vi "Post-Build Action.vi"(5 "Files Generated by Build":path[](array[path]), 6 "Top Level/Always Included VIs":path[](array[path]), 7 "Destination Path":path, 8 "error in":errorcluster, 9 "Target Name":string, 10 "Build Specification Name":string, 11 "Project Path":path) -> (0 "error out":errorcluster)   [LabVIEW 2026]
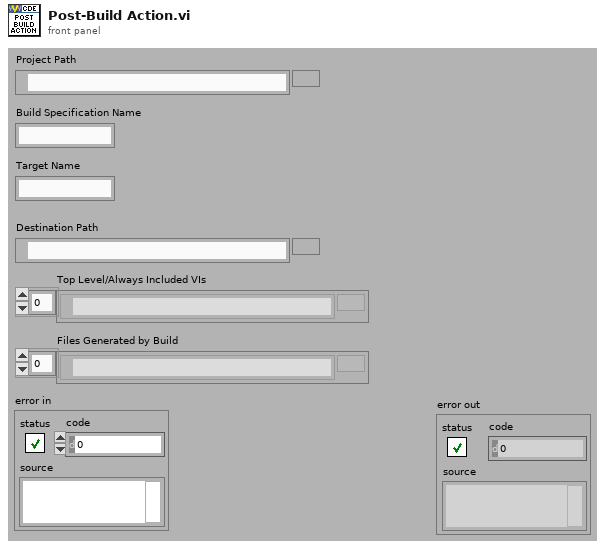
[diagram p1: front panel]
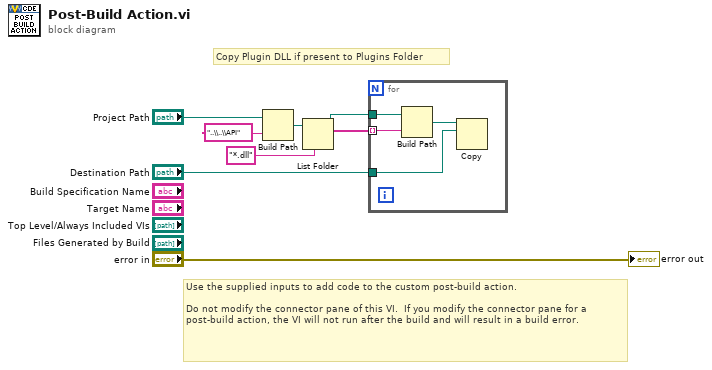
[diagram p0: block diagram]
diagram:
  # "Copy Plugin DLL if present to Plugins Folder"
  # "Use the supplied inputs to add code to the custom post-build action.\n\nDo not modify the connector pane of this VI.  If you modify the connector pane for a post-build action, the VI will not run after the build and will result in a build error."
  n1 = Build Path(base path="Project Path", name or relative path="..\\..\\API") -> (appended path=w4:path)
  n2 = List Folder(path=w4, pattern="*.dll") -> (path out=w3:path, filenames=w2:string[])  [unwired: 2 in, 2 out]
  n3 = for {
    tunnel: w3 -> [w12]
    tunnel: w2 -> [w11] mode=indexing
    tunnel: "Destination Path" -> [w9]
    n4 = Build Path(base path=w12, name or relative path=w11) -> (appended path=w10:path)
    n5 = Copy(10:w9, 11:w10) -> ()  [unwired: 3 in, 3 out]
  }
  "error out" <- "error in"
